vi "formatAmplifierOutputs.vi"(8 "error in (no error)":errorcluster, 11 "ILC in":refnum<class "ILC.lvclass">) -> (0 "error out":errorcluster, 2 "formattedOutputData":string, 3 "ILC out":refnum<class "ILC.lvclass">)   [LabVIEW 2015, in "ILCCommon.lvlib" / "ILC.lvclass"]
uses:
  <userlib>/Common/ILC/ILC/ILC.lvclass
  <userlib>/Common/ILC/ILC/ILC.lvclass/ILC.ctl
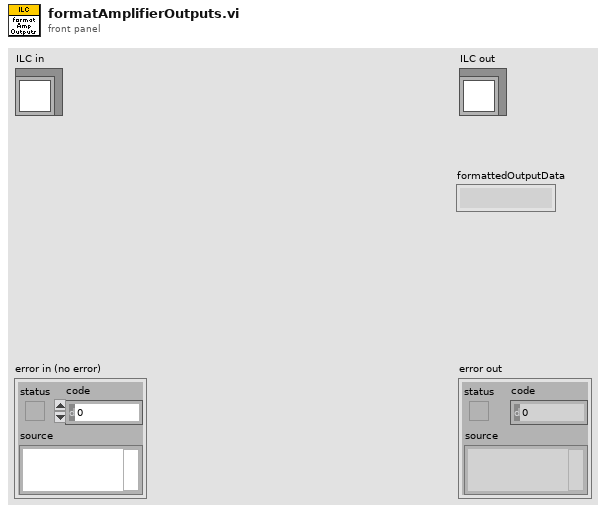
[diagram p1: front panel]
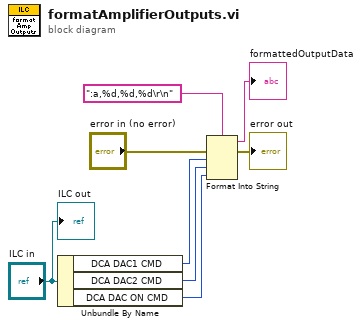
[diagram p0: block diagram]
diagram:
  n1 = Unbundle By Name("ILC in") -> ("DCA DAC1 CMD"=w4:u16, "DCA DAC2 CMD"=w3:u16, "DCA DAC ON CMD"=w2:u16)
  n2 = Format Into String(format string=":a,%d,%d,%d\r\n", error in="error in (no error)", w4, w3, w2) -> (resulting string=→"formattedOutputData":string, error out=→"error out":errorcluster)  [unwired: 1 in]
  "ILC out" <- "ILC in"
